vi "pid.vi"(7 "LVWSR":refnum<class "Web Request.lvclass">) -> ()   [LabVIEW 2014]
uses:
  <vilib>/wsapi/Web Request.lvclass
  Controller/Messages/Update TEC PID/Update TEC PID.lvclass
  Controller/Messages/Pack Message for Shipping/Pack Message for Shipping .lvclass
  Controller/Messages/Update TEC PID/Update TEC PID.lvclass/Update TEC PID.ctl
  Controller/Messages/Pack Message for Shipping/Pack Message for Shipping .lvclass/Pack Message for Shipping .ctl
  Controller/Messages/Update TEC PID/Write ctl.vi
  Controller/Messages/Pack Message for Shipping/Write enqueuer.vi
  Controller/Messages/Pack Message for Shipping/Write Message.vi
  Controller/Controller.lvclass
panel:
  in  "PID":string
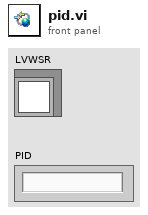
[diagram p1: front panel]
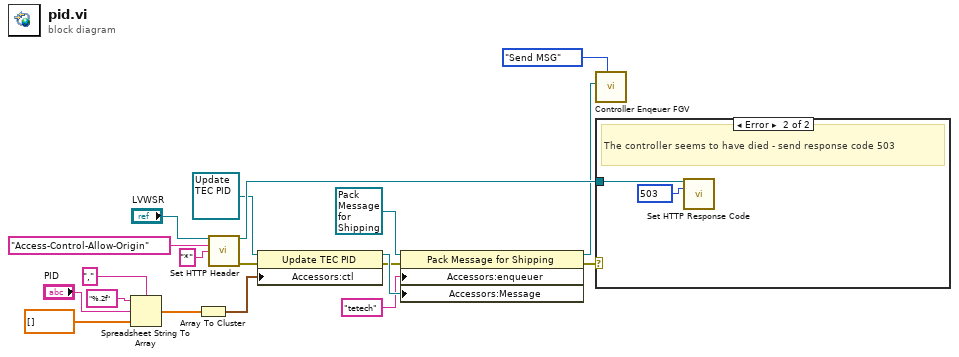
[diagram p0: block diagram]
diagram:
  n1 = Spreadsheet String To Array(delimiter (Tab)=",", format string="%.2f", spreadsheet string="PID", array type (2D Dbl)=dbl[] []) -> (array=w11:dbl[])
  n2 = Array To Cluster(array=w11) -> (cluster=w9:cluster{"[0]":dbl, "[1]":dbl, "[2]":dbl})
  n3 = call <vilib>:"Set HTTP Header.vi"("LabVIEW Web Service Request"="LVWSR", "header"="Access-Control-Allow-Origin", "header value"="*") -> ("LabVIEW Web Service Request out"=w16:refnum<class "Web Request.lvclass">, "error out"=w3:errorcluster)  [unwired: 11 in]
  n4 = property class="Update TEC PID"(reference=refnum<class "Update TEC PID.lvclass"> refnum ("Controller:Update TEC PID"), error in=w3, "Accessors:ctl"=w9) -> (reference out=w7:refnum<class "Update TEC PID.lvclass">, error out=w2:errorcluster)
  n5 = property class="Pack Message for Shipping"(reference=refnum<class "Pack Message for Shipping .lvclass"> refnum ("Controller:Pack Message for Shipping"), error in=w2, "Accessors:enqueuer"="tetech" ("enqueuer"), "Accessors:Message"=w7) -> (reference out=w5:refnum<class "Pack Message for Shipping .lvclass">, error out=w1:errorcluster)
  n6 = call "Controller Enqeuer FGV.vi"("State"=enum16{"Store", "Send MSG"}."Send MSG", "MSG"=w5) -> ()  [unwired: 9 in, 1 out]
  n7 = case shown="Error" w1 {
    tunnel: w16 -> [_ w20]
    frame No Error {
    }
    frame Error {
      w21 = 503 items=["100"=100, "101"=101, "200"=200, "201"=201, "202"=202, "203"=203, "204"=204, "205"=205, "206"=206, "300"=300, "301"=301, "302"=302, "303"=303, "304"=304, "305"=305, "306"=306, "307"=307, "400"=400, "401"=401, "402"=402, "403"=403, "404"=404, "405"=405, "406"=406, "407"=407, "408"=408, "409"=409, "410"=410, "411"=411, "412"=412, "413"=413, "414"=414, "415"=415, "416"=416, "417"=417, "500"=500, "501"=501, "502"=502, "503"=503, "504"=504, "505"=505] ("response code (200)")
      # "The controller seems to have died - send response code 503"
      n8 = call <vilib>:"Set HTTP Response Code.vi"("LabVIEW Web Service Request"=w20, "response code (200)"=w21) -> ()  [unwired: 12 in, 2 out]
    }
  }
